vi "Calculate dt loss.vi"(0 "No. of Steps":dbl, 5 "Floor(No.ofSteps)":dbl, 7 "Minimum Sequence Delta (S)":dbl, 13 "No. of steps is greater than 0?":bool) -> (4 "Minimum Sequence Delta (S)":dbl format="%#_15g")   [LabVIEW 2024, in "devicePowerSequencerCoreLogic.lvlib"]
uses:
  devicePowerSequencerCoreLogic.lvlib
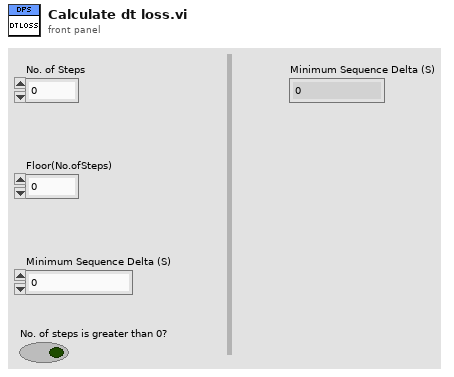
[diagram p1: front panel]
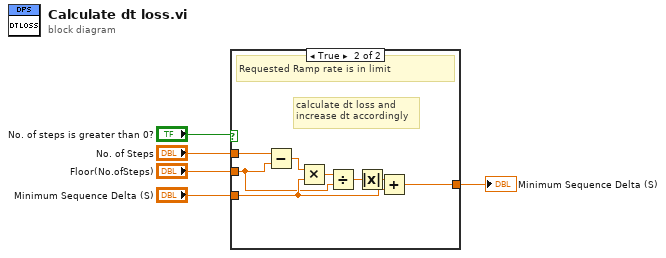
[diagram p0: block diagram]
diagram:
  n1 = case shown="True" "No. of steps is greater than 0?" {
    tunnel: "No. of Steps" -> [_ w14]
    tunnel: "Minimum Sequence Delta (S)" -> [w6 w11]
    tunnel: [w6 w9] -> w1
    tunnel: "Floor(No.ofSteps)" -> [_ w8]
    frame False {
      # "Requested Ramp rate is not in limit"
    }
    frame True {
      # "calculate dt loss and\nincrease dt accordingly"
      # "Requested Ramp rate is in limit"
      n2 = Subtract(x=w14, y=w8) -> (x-y=w10:dbl)
      n3 = Multiply(x=w10, y=w11) -> (x*y=w12:dbl)
      n4 = Divide(x=w12, y=w8) -> (x/y=w13:dbl)
      n5 = Absolute Value(x=w13) -> (abs(x)=w7:dbl)
      n6 = Add(x=w7, y=w11) -> (x+y=w9:dbl)
    }
  }
  "Minimum Sequence Delta (S)" <- w1
